vi "Menu.DisableAll.vi"(8 "error in (no error)":errorcluster, 11 "Menu in":refnum<k9>) -> (0 "error out":errorcluster)   [LabVIEW 2015, in "Multihead GUI.lvlib"]
uses:
  Multihead GUI.lvlib
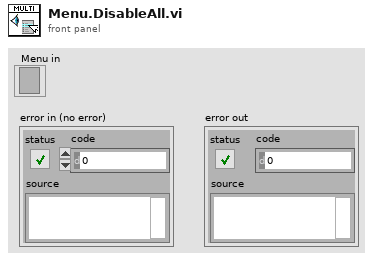
[diagram p1: front panel]
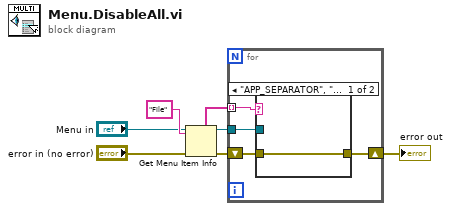
[diagram p0: block diagram]
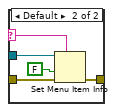
[diagram p2: hidden frame]
diagram:
  n1 = Get Menu Item Info(7:"File" ("item tag"), 8:"error in (no error)", 11:"Menu in") -> (0:w2:errorcluster, 3:w3:refnum<k9>, 5:w5:string[])  [unwired: 4 out]
  n2 = for {
    tunnel: w3 -> [w10]
    tunnel: w5 -> [w8] mode=indexing
    shift-right: [w9] -> w7
    shift-left: w2 -> [w11]
    n3 = case shown="\"APP_SEPARATOR\", \"Macro.Exit\"" w8 {
      selector: w8 -> [_ w13]
      tunnel: w11 -> [w12 w17]
      tunnel: w10 -> [_ w16]
      tunnel: [w12 w14] -> w9
      frame "APP_SEPARATOR", "Macro.Exit" {
      }
      frame Default {
        n4 = Set Menu Item Info(7:w13, 8:w17, 9:FALSE ("enabled"), 11:w16) -> (0:w14:errorcluster)  [unwired: 3 in, 1 out]
      }
    }
  }
  "error out" <- w7
